vi "GetHTTPStats.vi"(8 "error in (no error)":errorcluster, 11 "ClashRoyale in":refnum<class "StashRoyale.lvclass">) -> (0 "error out":errorcluster, 3 "ClashRoyale out":refnum<class "StashRoyale.lvclass">)   [LabVIEW 2020, in "StashRoyale.lvclass"]
uses:
  StashRoyale.lvclass
  StashRoyale.lvclass/StashRoyale.ctl
  <vilib>/httpClient/LabVIEWHTTPClient.lvlib
  <vilib>/addons/Tools/Unicode/UTF8 Tools.lvlib
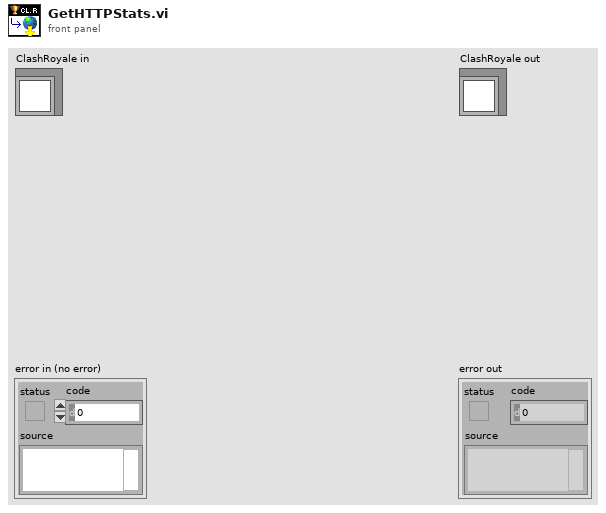
[diagram p1: front panel]
types:
  T1 = typedef "LabVIEWHTTPClient.lvlib/ClientHandle.ctl" = refnum<k1>
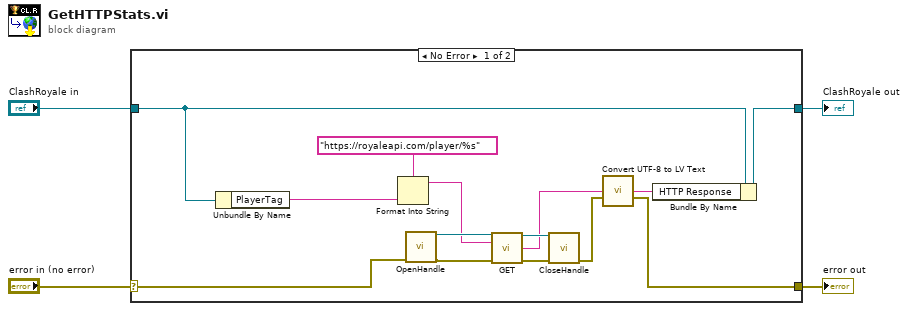
[diagram p0: block diagram]
diagram:
  n1 = case shown="No Error" "error in (no error)" {
    selector: "error in (no error)" -> [w13 w20]
    tunnel: [w5 w20] -> w3
    tunnel: [w8 w19] -> w1
    tunnel: "ClashRoyale in" -> [w10 w19]
    frame No Error {
      n2 = Unbundle By Name(w10) -> ("PlayerTag"=w9:string)
      n3 = Format Into String(format string="https://royaleapi.com/player/%s" ("url"), w9) -> (resulting string=w11:string)  [unwired: 2 in, 1 out]
      n4 = call <vilib>:"OpenHandle.vi"("error in (no error)"=w13) -> ("client handle out"=w18:T1, "error out"=w17:errorcluster)  [unwired: 13 in]
      n5 = call <vilib>:"GET.vi"("client handle"=w18, "url"=w11, "error in (no error)"=w17) -> ("client handle out"=w16:T1, "body"=w14:string, "error out"=w15:errorcluster)  [unwired: 9 in, 1 out]
      n6 = call <vilib>:"CloseHandle.vi"("client handle"=w16, "error in (no error)"=w15) -> ("error out"=w6:errorcluster)  [unwired: 13 in]
      n7 = call <vilib>:"Convert UTF-8 to LV Text.vi"("UTF-8 Text"=w14, "error in"=w6) -> ("LV Text"=w7:string, "error out"=w5:errorcluster)  [unwired: 12 in]
      n8 = Bundle By Name(cluster=w10, "HTTP Response"=w7) -> (w8:refnum<class "StashRoyale.lvclass">)
    }
    frame Error {
    }
  }
  "error out" <- w3
  "ClashRoyale out" <- w1
